vi "CSTK_Enum_Creator_CreateEnum.vi"(8 "错误输入（无错误）":errorcluster, 10 "样式":u32, 11 "VI输入":refnum<vi>) -> (0 "错误输出":errorcluster, 2 "Enum输出":refnum<vi>, 3 "VI输出":refnum<vi>)   [LabVIEW 2015, in "CSTK_Enum Creator.lvlib"]
uses:
  CSTK_Enum Creator.lvlib
  <vilib>/Utility/miscctls.llb/LVPointTypeDef.ctl
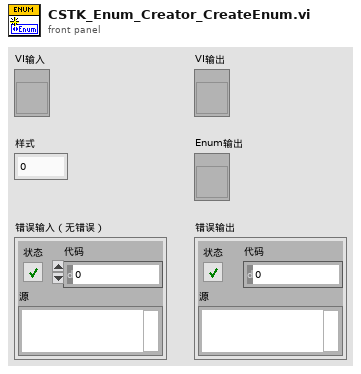
[diagram p1: front panel]
types:
  T1 = typedef "LVPointTypeDef.ctl" = cluster{"Horizontal":i16, "Vertical":i16}
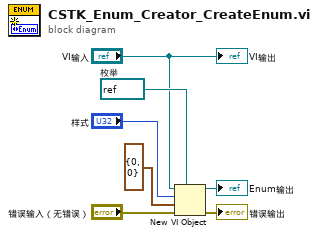
[diagram p0: block diagram]
diagram:
  w2 = refnum<vi> refnum  # 枚举
  n1 = New VI Object(vi object class=w2, owner refnum="VI输入", style="样式", position/next to=T1 {"Horizontal"=0, "Vertical"=0} ("位置"), 8:"错误输入（无错误）") -> (object refnum=→"Enum输出":refnum<vi>, 0:→"错误输出":errorcluster)  [unwired: 3 in]
  "VI输出" <- "VI输入"
